vi "subConvertValueToNameAndPath.vi"(7 "RelativeToProject":bool, 9 "Project path":path, 10 "TargetName":string, 11 "Value":string) -> (1 "Path":path, 3 "Name":string)   [LabVIEW 2019, in "SolutionBuilder.lvlib" / "SolutionBuilder.lvclass"]
uses:
  SolutionBuilder.lvclass
  <vilib>/regexp/Match Regular Expression.xnode
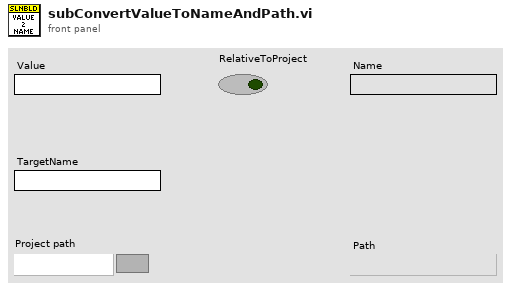
[diagram p1: front panel]
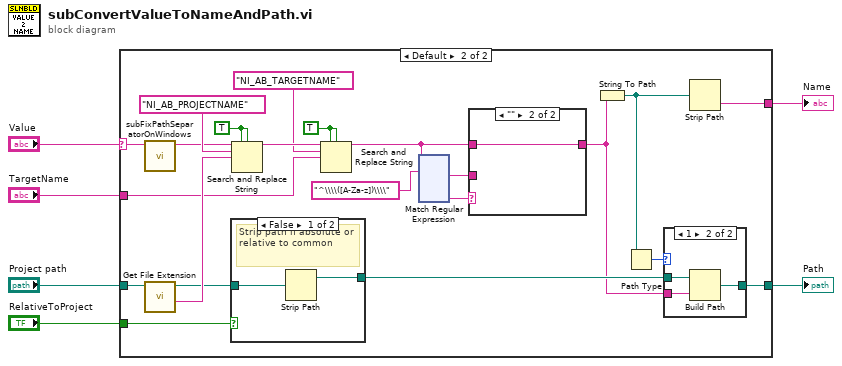
[diagram p0: block diagram]
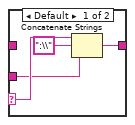
[diagram p4: hidden frame]
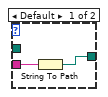
[diagram p5: hidden frame]
diagram:
  n1 = case shown="Default" "Value" {
    selector: "Value" -> [_ w11]
    tunnel: [_ w26] -> w3
    tunnel: "Project path" -> [_ w25]
    tunnel: [_ w22] -> w5
    tunnel: "TargetName" -> [_ w12]
    tunnel: "RelativeToProject" -> [_ w7]
    frame "" {
    }
    frame Default {
      w16 = TRUE ("replace all? (F)")
      w28 = TRUE ("replace all? (F)")
      n2 = call "subFixPathSeparatorOnWindows.vi"("Value"=w11) -> ("fixed path"=w10:string)  [unwired: 10 in]
      n3 = call <vilib>:"Get File Extension.vi"("file"=w25) -> ("filename without extension"=w24:string, "dup file"=w23:path)  [unwired: 6 in, 3 out]
      n4 = case shown="False" w7 {
        tunnel: w23 -> [w30 w31]
        tunnel: [w29 w31] -> w21
        frame False {
          # "Strip path if absolute or relative to common"
          n5 = Strip Path(path=w30) -> (stripped path=w29:path)  [unwired: 1 out]
        }
        frame True {
          # "Do not strip path if relative to project"
        }
      }
      n6 = Search and Replace String(replace all?=w28, case sensitive?=w28, input string=w10, search string="NI_AB_PROJECTNAME", replace string=w24) -> (result string=w15:string)  [unwired: 3 in, 3 out]
      n7 = Search and Replace String(replace all?=w16, case sensitive?=w16, input string=w15, search string="NI_AB_TARGETNAME", replace string=w12) -> (result string=w14:string)  [unwired: 3 in, 3 out]
      n8 = xnode "Match Regular Expression"("input string"=w14, "regular expression"="^\\\\([A-Za-z])\\\\") -> ("after match"=w18:string, "submatch 1"=w17:string)  [unwired: 4 in, 4 out]
      n9 = case shown="\"\"" w17 {
        selector: w17 -> [w151 _]
        tunnel: [w149 w152] -> w19
        tunnel: w14 -> [_ w152]
        tunnel: w18 -> [w148 _]
        frame Default {
          n10 = Concatenate Strings(w151, ":\\" ("string"), w148) -> (w149:string)
        }
        frame "" {
        }
      }
      n11 = String To Path(string=w19) -> (path=w9:path)
      n12 = Path Type(1:w9) -> (0:w8:i16)
      n13 = case shown="1" w8 {
        tunnel: w21 -> [_ w157]
        tunnel: w19 -> [w154 w156]
        tunnel: [w153 w155] -> w22
        frame Default {
          n14 = String To Path(string=w154) -> (path=w153:path)
        }
        frame 1 {
          n15 = Build Path(base path=w157, name or relative path=w156) -> (appended path=w155:path)
        }
      }
      n16 = Strip Path(path=w9) -> (name=w26:string)  [unwired: 1 out]
    }
  }
  "Path" <- w5
  "Name" <- w3
